vi "Untitled 1.vi"() -> ()   [LabVIEW 2013]
uses:
  <vilib>/picture/picture.llb/Draw True-Color Pixmap.vi
  <vilib>/addons/Modulation/Digital/General/MT Generate Bits (Galois, PN Order).vi
  <vilib>/addons/Modulation/Digital/General/MT Generate PSK System Parameters(M).vi
  <vilib>/addons/Modulation/Digital/General/MT Generate PSK Synchronization Parameters (bit array).vi
  <vilib>/addons/Modulation/Digital/General/MT Format Eye Diagram (complex).vi
  <vilib>/Utility/file.llb/Write To Spreadsheet File (I64).vi
  <vilib>/addons/Modulation/niDMT.lvlib
panel:
  in  "file path (dialog if empty)":path
  in  "path to JPEG file":path
  out "measurements":T1 {"phase offset (deg)" format="%.2f"; "frequency drift (Hz)" format="%.2f"; "frequency offset (Hz)" format="%.2f"}
  out "LED output":cluster{bool[], bool[]}
  in  "Tab Control":enum32{"Page 1", "Page 2", "Page 3"}(tab)
  out "Waveform Graph 2":cluster{"t0":dbl, "dt":dbl, "Y":dbl[]}[](graph)
  out "XY Graph":T2(graph)
  out "recovered":picture
  out "original":picture
  out "Waveform Graph":cluster{"t0":dbl, "dt":dbl, "Y":dbl[]}(graph)
  in  "stop":bool
  out "error out":errorcluster
  out "sync found index (symbols)":dbl format="%.4f"
  in  "Eb/N0 (10 dB)":dbl=10.0 caption="Eb/N0"
  in  "modulation type":T3(ring)
  in  "pulse shaping filter (none)":T4(ring)
  in  "M-FSK (2)":i32=2
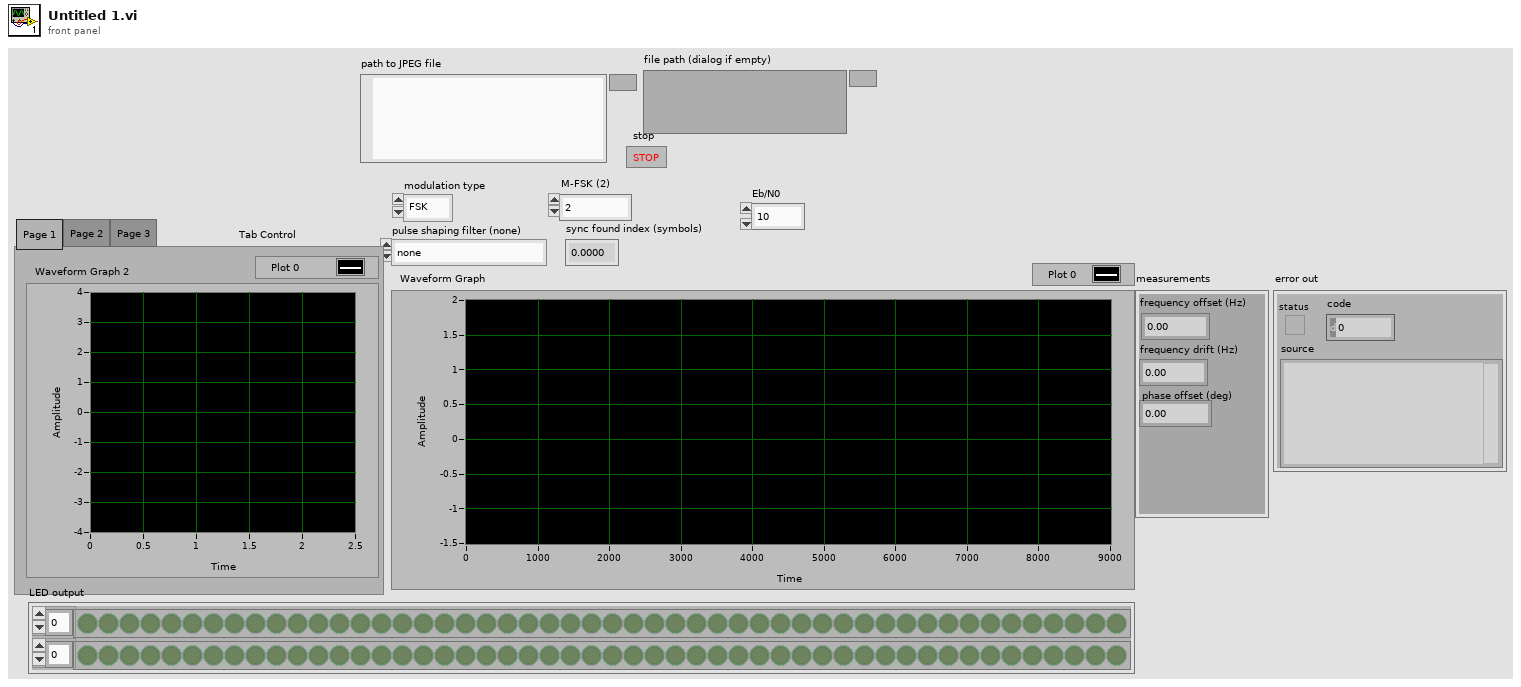
[diagram p1: front panel]
types:
  T1 = cluster{"frequency offset (Hz)":dbl, "frequency drift (Hz)":dbl, "phase offset (deg)":dbl}
  T2 = cluster{"constellation":dbl[], "oversampled data":dbl[]}[]
  T3 = enum16{"FSK", "PSK", "QAM", "MSK", "PAM", "ASK", "CPM"}
  T4 = enum16{"none", "Raised Cosine", "Root Raised Cos", "Gaussian"}
  T5 = typedef "imagedata.ctl" = cluster{"image type":i32, "image depth":i32, "image":u8[], "mask":u8[], "colors":u32[], "Rectangle":cluster{"left":i16, "top":i16, "right":i16, "bottom":i16}}
  T6 = cluster{"samples per symbol (16)":i32, "symbol map":cdb[], "differential PSK":enum16{"disable", "enable"}, "PSK type":u16}
  T7 = typedef "niAMT.lvlib/Complex Data Waveform.ctl" = cluster{"t0":dbl, "dt":dbl, "Y":cdb[]}
  T8 = cluster{"expected sync location (symbols)":i32, "sync sequence":cdb[], "sync location uncertainty (symbols)":i32, "sync indent (symbols)":i32}
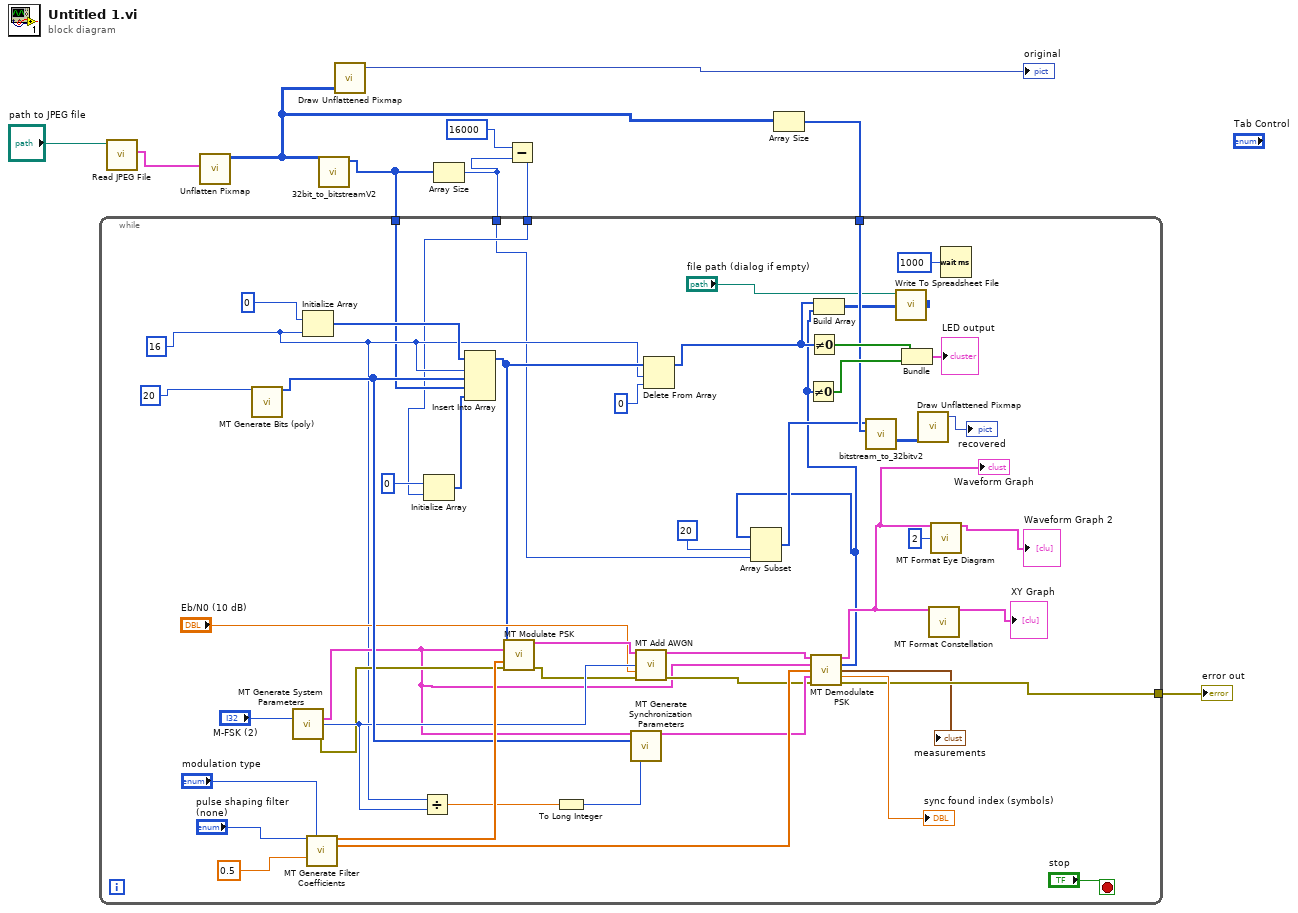
[diagram p0: block diagram]
diagram:
  n1 = call <vilib>:"Read JPEG File.vi"("path to JPEG file"="path to JPEG file") -> ("image data"=w8:T5)  [unwired: 8 in, 2 out]
  n2 = call <vilib>:"Unflatten Pixmap.vi"("image data"=w8) -> ("24-bit pixmap"=w2:u32[][])  [unwired: 4 in, 6 out]
  n3 = call "32bit_to_bitstreamV2.vi"("24-bit pixmap"=w2) -> ("Bitstream with Guard"=w4:u8[])  [unwired: 7 in, 1 out]
  n4 = call-poly <vilib>:"Draw Unflattened Pixmap.vi"("data (RGB format)"=w2) -> ("new picture"=→"original":picture)  [unwired: 8 in]
  n5 = Array Size(array=w4) -> (size(s)=w1:i32)
  n6 = Subtract(x=16000, y=w1) -> (x-y=w5:i32)
  n7 = Array Size(array=w2) -> (size(s)=w3:i32[])
  n8 = while {
    tunnel: [w36] -> w10
    tunnel: w4 -> [w25]
    tunnel: w5 -> [w23]
    tunnel: w3 -> [w21]
    tunnel: w1 -> [w19]
    stop <- "stop" stop-if-true
    w26 = 16
    n9 = call-poly <vilib>:"MT Generate Bits (poly).vi"("total bits (128)"=20) -> ("output bit stream"=w45:i8[])  [unwired: 12 in, 2 out]
    n10 = call-poly <vilib>:"MT Generate System Parameters.vi"("M-PSK (4)"="M-FSK (2)") -> ("PSK system parameters"=w30:T6, "bits per symbol"=w44:i32, "error out"=w41:errorcluster)  [unwired: 12 in]
    n11 = Initialize Array(0, w26) -> (w59:i32[])
    n12 = call <vilib>:"MT Generate Filter Coefficients.vi"("pulse shaping filter (none)"="pulse shaping filter (none)", "modulation type"="modulation type", "filter parameter"=0.5) -> ("pulse shaping filter coefficients"=w50:dbl[], "matched filter coefficients"=w49:dbl[])  [unwired: 10 in, 1 out]
    n13 = Divide(x=w26, y=w44) -> (x/y=w43:dbl)
    n14 = Initialize Array(i8 0 ("element"), w23) -> (w22:i8[])
    n15 = Insert Into Array(array=w59, index=w26, new element #1=w45, new element #2=w25, new element #3=w22) -> (w27:i32[])
    n16 = call <vilib>:"MT Modulate PSK.vi"("input bit stream"=w27, "PSK system parameters"=w30, "pulse shaping filter coefficients"=w50, "error in (no error)"=w41) -> ("output complex waveform"=w46:T7, "error out"=w40:errorcluster)  [unwired: 9 in, 1 out]
    n17 = To Long Integer(number=w43) -> (32bit integer=w42:i32)
    n18 = call-poly <vilib>:"MT Generate Synchronization Parameters.vi"("PSK system parameters"=w30, "sync bits"=w45, "expected sync location (symbols)"=w42) -> ("PSK synchronization parameters"=w48:T8)  [unwired: 11 in, 1 out]
    n19 = call <vilib>:"MT Add AWGN.vi"("input complex waveform"=w46, "bits per symbol (1)"=w44, "Eb/N0 (10 dB)"="Eb/N0 (10 dB)", "error in (no error)"=w40) -> ("output complex waveform"=w47:T7, "error out"=w39:errorcluster)  [unwired: 9 in, 1 out]
    n20 = Delete From Array "Delete From Array"(array=w27, length=w26, index=0) -> (array with subset deleted=w14:i32[])  [unwired: 1 out]
    n21 = Not Equal To 0?(x=w14) -> (x != 0?=w56:bool[])
    n22 = call <vilib>:"MT Demodulate PSK.vi"("input complex waveform"=w47, "PSK system parameters"=w30, "matched filter coefficients"=w49, "synchronization parameters"=w48, "error in (no error)"=w39) -> ("recovered complex waveform"=w33:T7, "output bit stream"=w13:i8[], "measurements"=→"measurements":T1, "sync found index (symbols)"=→"sync found index (symbols)":dbl, "error out"=w36:errorcluster)  [unwired: 6 in]
    "Waveform Graph" <- w33
    n23 = Array Subset(array=w13, index=20, length=w19) -> (w18:i8[])
    n24 = Not Equal To 0?(x=w13) -> (x != 0?=w55:bool[])
    n25 = Build Array(w14, w13) -> (w12:i32[][])
    n26 = call "bitstream_to_32bitv2.vi"("JPG Size"=w21, "Bitstream Input"=w18) -> ("2D JPG Array"=w15:u32[][])  [unwired: 8 in, 1 out]
    n27 = call-poly <vilib>:"Write To Spreadsheet File.vi"("2D data"=w12, "file path (dialog if empty)"="file path (dialog if empty)") -> ()  [unwired: 6 in, 1 out]
    n28 = Bundle(w56, w55) -> (→"LED output":cluster{bool[], bool[]})  [unwired: 1 in]
    n29 = call-poly <vilib>:"Draw Unflattened Pixmap.vi"("data (RGB format)"=w15) -> ("new picture"=→"recovered":picture)  [unwired: 8 in]
    n30 = call <vilib>:"MT Format Constellation.vi"("waveform"=w33) -> ("constellation graph"=→"XY Graph":T2)  [unwired: 13 in, 1 out]
    n31 = call-poly <vilib>:"MT Format Eye Diagram.vi"("waveform"=w33, "eye length"=2) -> ("eye diagram"=→"Waveform Graph 2":cluster{"t0":dbl, "dt":dbl, "Y":dbl[]}[])  [unwired: 12 in, 1 out]
    n32 = Wait (ms)(milliseconds to wait=u32 1000) -> ()  [unwired: 1 out]
  }
  "error out" <- w10
